vi "calculateImpedance.vi"(9 "Vmeas":dbl, 10 "Vb":dbl, 11 "V":dbl) -> (3 "Z":dbl)   [LabVIEW 2011]
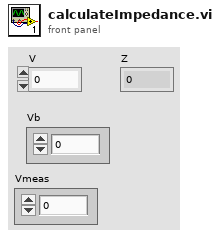
[diagram p1: front panel]
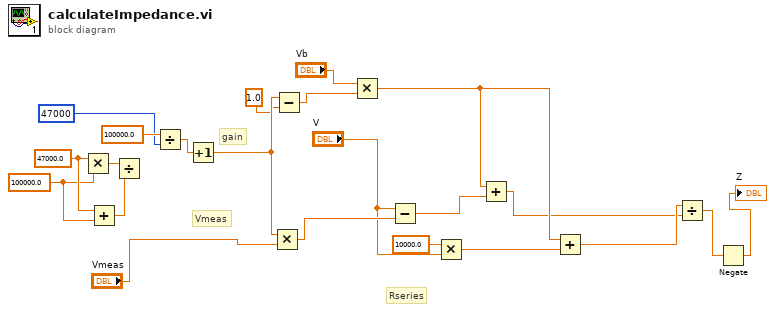
[diagram p0: block diagram]
diagram:
  w19 = 100000.0 ("y")
  w20 = 47000.0 ("x")
  # "Rseries"
  # "Vmeas"
  # "gain"
  n1 = Multiply(x=w20, y=w19) -> (x*y=w21:dbl)
  n2 = Add(x=w20, y=w19) -> (x+y=w18:dbl)
  n3 = Divide(x=w21, y=w18) -> ()  [unwired: 1 out]
  n4 = Divide(x=100000.0, y=47000) -> (x/y=w16:dbl)
  n5 = Increment(x=w16) -> (x+1=w4:dbl)
  n6 = Multiply(x=w4, y="Vmeas") -> (x*y=w12:dbl)
  n7 = Subtract(x=w4, y=1.0 ("x")) -> (x-y=w14:dbl)
  n8 = Multiply(x="Vb", y=w14) -> (x*y=w9:dbl)
  n9 = Subtract(x="V", y=w12) -> (x-y=w10:dbl)
  n10 = Multiply(x=10000.0, y="V") -> (x*y=w13:dbl)
  n11 = Add(x=w9, y=w10) -> (x+y=w7:dbl)
  n12 = Add(x=w9, y=w13) -> (x+y=w8:dbl)
  n13 = Divide(x=w8, y=w7) -> (x/y=w6:dbl)
  n14 = Negate(x=w6) -> (-x=→"Z":dbl)
